vi "Init Non-SD Page.vi"(8 "error in (no error)":errorcluster, 10 "SubPanel Ref":refnum<vi>, 11 "Node Ptr In":T1 format="%.0x") -> (0 "error out":errorcluster, 2 "SD Module":refnum<class "SD Module.lvclass">, 3 "Node Ptr Out":T1 format="%.0x", 5 "SubPanel Command":refnum<user-event>)   [LabVIEW 2017, in "Modules.lvlib" / "SD Module.lvclass"]
uses:
  SD Module.lvclass
  <vilib>/NI Veristand/Custom Device API/Custom Device Item Ref.ctl
  RSI Module/SubPanel Command.ctl
  RSI Module/RSI Module.lvclass
  <vilib>/NI Veristand/Custom Device API/Custom Device API.lvlib
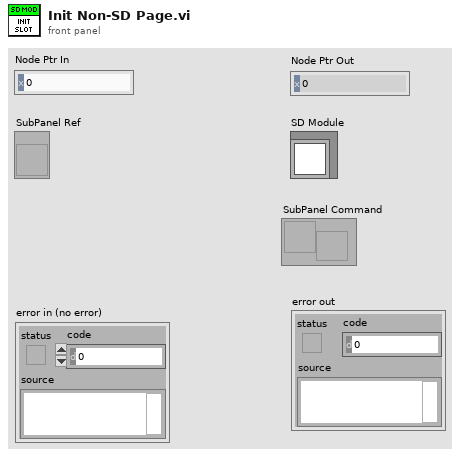
[diagram p1: front panel]
types:
  T1 = typedef "Custom Device API.lvlib/Custom Device Item Ref.ctl" = u64
  T2 = typedef "Modules.lvlib/RSI Module.lvclass/SubPanel Command.ctl" = enum16{"Stop"}
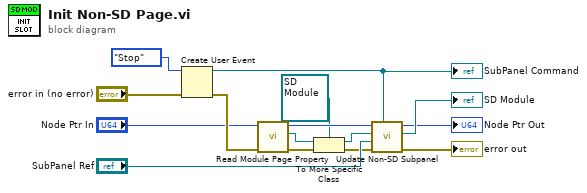
[diagram p0: block diagram]
diagram:
  n1 = Create User Event(user event datatype=SubPanel_Command."Stop" ("SubPanel Command"), error in="error in (no error)") -> (user event=w11:refnum<user-event>, error out=w14:errorcluster)
  "SubPanel Command" <- w11
  n2 = call "Read Module Page Property.vi"("error in (no error)"=w14, "Node Ptr In"="Node Ptr In") -> ("error out"=w2:errorcluster, "RSI Module"=w4:refnum<class "RSI Module.lvclass">, "Node Ptr Out"=w15:T1)  [unwired: 7 in]
  n3 = To More Specific Class(target class=refnum<class "SD Module.lvclass"> refnum ("Modules.lvlib:SD Module.lvclass"), reference=w4, error in=w2) -> (specific class reference=w3:refnum<class "SD Module.lvclass">, error out=w1:errorcluster)
  n4 = call "Update Non-SD Subpanel.vi"("SubPanel Command"=w11, "error in (no error)"=w1, "SubPanel Ref"="SubPanel Ref", "SD Module in"=w3, "Node Ptr In"=w15) -> ("error out"=→"error out":errorcluster, "SD Module out"=→"SD Module":refnum<class "SD Module.lvclass">, "Node Ptr Out"=→"Node Ptr Out":T1)  [unwired: 4 in]
